vi "gScript Pattern Recognition Tuner.vi"() -> ()   [LabVIEW 2023]
doc: "Use this template to build a controller/worker design pattern. The controller loop always executes. It notifies one or more worker loops to execute their code. The worker loop(s) continue executing until they complete, then wait for another notification. Contrast this with the Producer/Consumer pattern in which the consumer loops execute only when they have data in their queue."
uses:
  find_patches parameters.ctl
  find_circles parameters.ctl
  find_rects_parameters.ctl
  find_template parameters.ctl
  Vision.lvlib
panel:
  in  "Fiducial ID":string
  out "Y Resolution":i32
  out "X Resolution":i32
  out "ROI":cluster{"width(mm)":dbl, "height(mm)":dbl} {"height(mm)" format="%#_3f"; "width(mm)" format="%#_3f"}
  in  "shrinkFactor":i32=4
  in  "Go Button":bool
  in  "Debug":bool
  in  "Field of View":cluster{"fieldOfViewX":sgl, "fieldOfViewY":sgl}={"fieldOfViewX"=1.4, "fieldOfViewY"=1.048}
  out "config lines":string
  out "Log":string
  in  "Results":T1(tab)
  out "Patches":T2(array[cluster])
  out "Circles":T3(array[cluster])
  out "rects":T4(array[cluster]) {"x" format="%#_3g"; "y" format="%#_3g"; "width" format="%#_3g"; "height" format="%#_3g"; "angle" format="%#_3g"; "image-x" format="%#_3g"; "image-y" format="%#_3g"}
  out "Matches":T5(array[cluster])
  in  "Sample Image":path
  out "Image":T6(plugin-control)
  in  "Parameters":T1(tab)
  in  "find_patches parameters":T7={"dilateSize"=6, "sizeMin"=0.1, "sizeMax"=0.3, "aspectRatioMin"=0.1, "aspectRatioMax"=1.1, "colorGroups"=2} {"sizeMin" step=0.05}
  in  "find_circles parameters":T8={"minRadius"=0.1, "maxRadius"=1.0, "houghGradientParam1"=100, "houghGradientParam2"=50}
  in  "find_rects parameters":T9={"nominalWidth"=1.0, "nominalHeight"=1.0, "tolerance"=0.5, "pointSelect"=4.0, "allowRotation"=FALSE}
  in  "find_template parameters":T10={"templateBlurFactor"=0, "minConcurrence"=0.0, "templatePath"="C:\\Users\\Caleb\\Desktop\\nebraska-silicon-lab\\pixel-gantry-control\\Example Project\\Data\\reference_images\\BBM_fid_template.png"}
  # "Tips:\n\n  -"
  # "Tips:\n\n  - minRadius & maxRadius\nare in mm"
  # "Tips:\n\n  - \n\npointSelect:\n  0: center\n  1: bottom-left corner\n  2: top-left corner\n  3: top-right corner\n  4: bottom-right corner"
  # "Tips:\n\n  -"
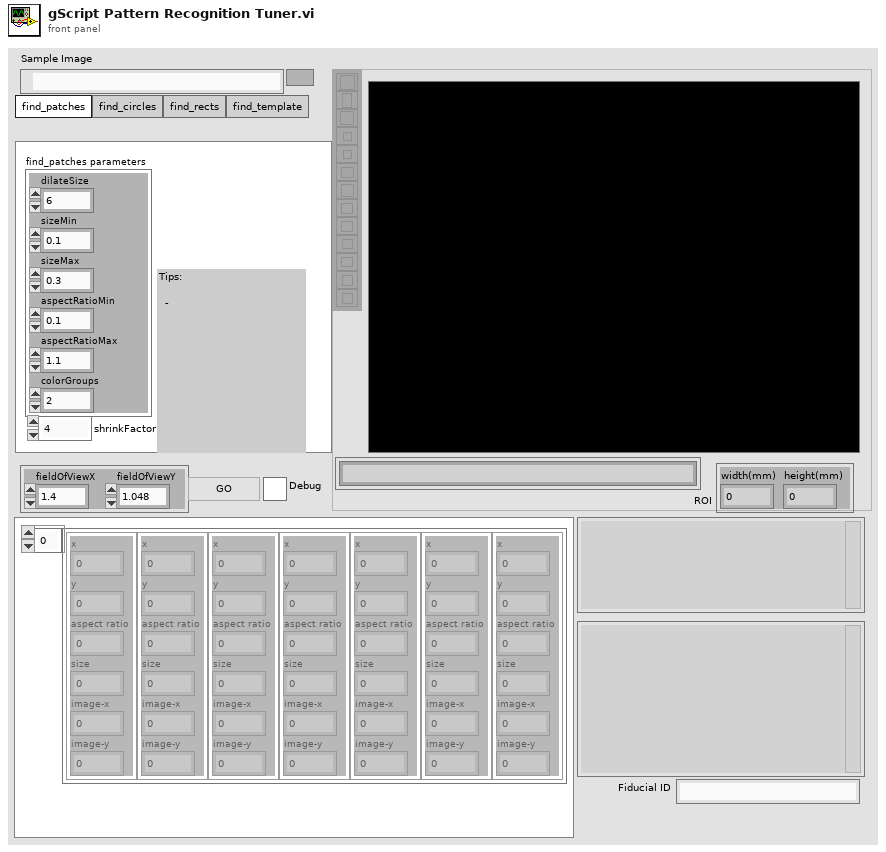
[diagram p1: front panel]
types:
  T1 = enum32{"find_patches", "find_circles", "find_rects", "find_template"}
  T2 = cluster{"x":dbl, "y":dbl, "aspect ratio":dbl, "size":dbl, "image-x":dbl, "image-y":dbl}[]
  T3 = cluster{"x":dbl, "y":dbl, "radius":dbl, "image-x":dbl, "image-y":dbl}[]
  T4 = cluster{"x":dbl, "y":dbl, "width":dbl, "height":dbl, "angle":dbl, "image-x":dbl, "image-y":dbl}[]
  T5 = cluster{"x":dbl, "y":dbl, "image-x":dbl, "image-y":dbl, "Concurrence":dbl}[]
  T6 = typedef "IMAQ Image.ctl" = refnum<image>
  T7 = typedef "Vision.lvlib/find_patches parameters.ctl" = cluster{"dilateSize":i32, "sizeMin":sgl, "sizeMax":sgl, "aspectRatioMin":sgl, "aspectRatioMax":sgl, "colorGroups":i32}
  T8 = typedef "Vision.lvlib/find_circles parameters.ctl" = cluster{"minRadius":sgl, "maxRadius":sgl, "houghGradientParam1":i32, "houghGradientParam2":i32}
  T9 = typedef "Vision.lvlib/find_rects_parameters.ctl" = cluster{"nominalWidth":sgl, "nominalHeight":sgl, "tolerance":sgl, "pointSelect":sgl, "allowRotation":bool}
  T10 = typedef "Vision.lvlib/find_template parameters.ctl" = cluster{"templateBlurFactor":i32, "minConcurrence":sgl, "templatePath":string}
  T11 = enum8{"Enabled", "Disabled", "Disabled and Grayed Out"}
  T12 = cluster{"Left":i32, "Top":i32, "Right":i32, "Bottom":i32}
  T13 = typedef "Image Type" = u32
  T14 = cluster{"Global Rectangle":i32[], "Contours":cluster{"Contour Type":u32, "ROI Type":u32, "Points":i32[]}[]}
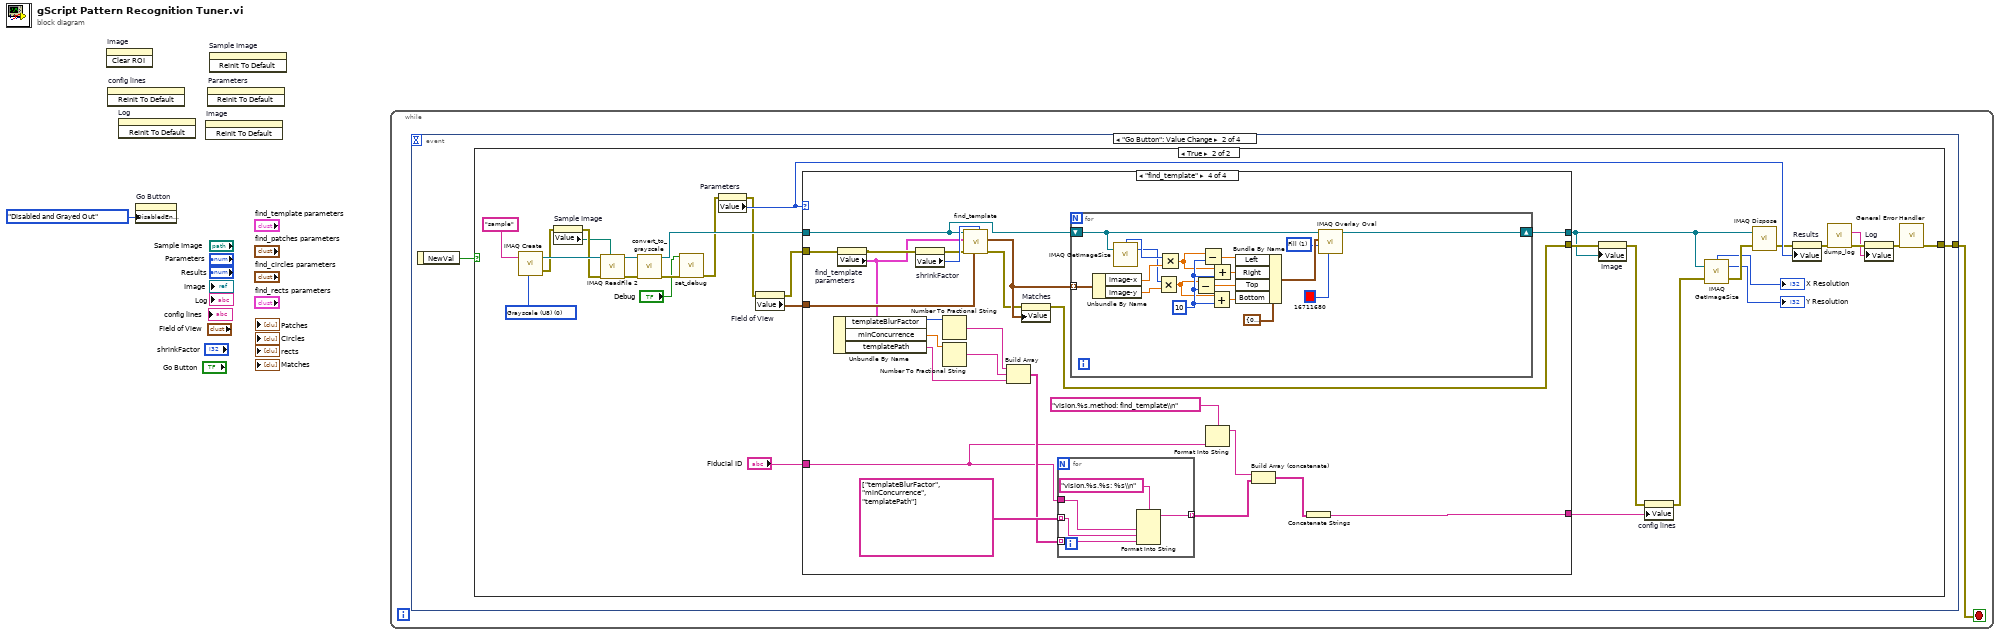
[diagram p0: block diagram]
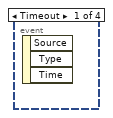
[diagram p2: hidden frame]
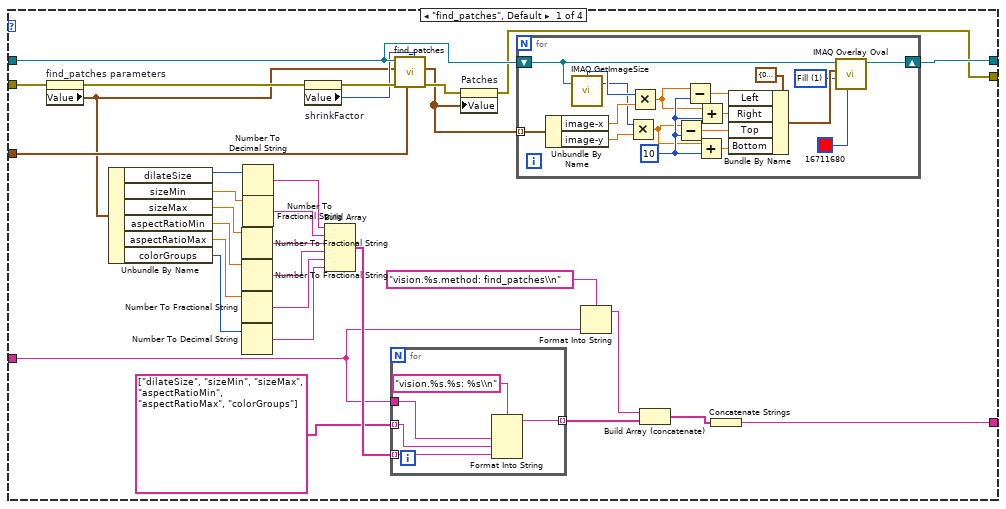
[diagram p4: hidden frame]
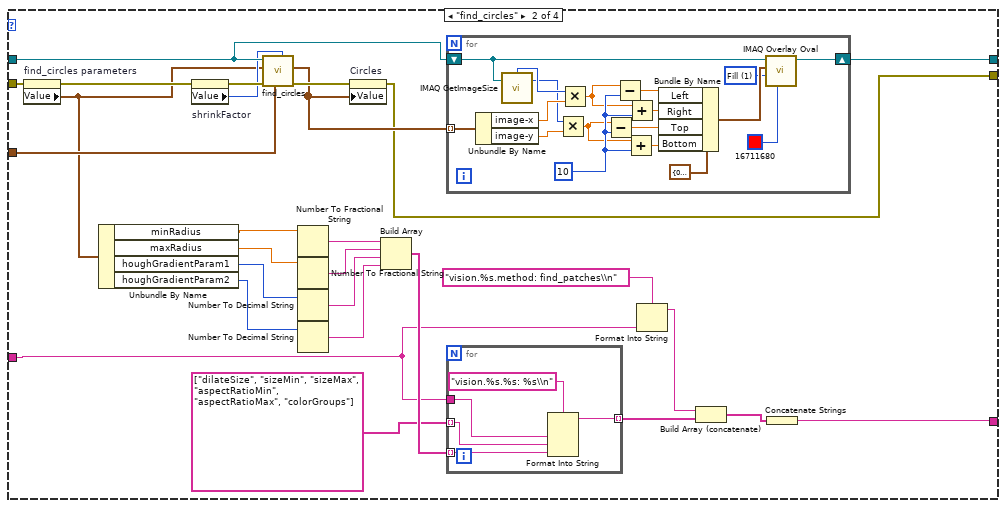
[diagram p5: hidden frame]
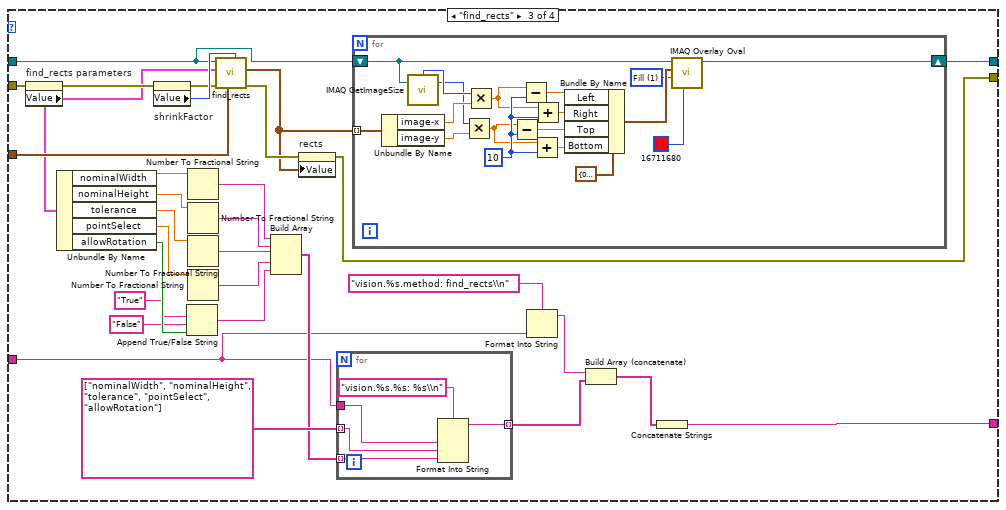
[diagram p6: hidden frame]
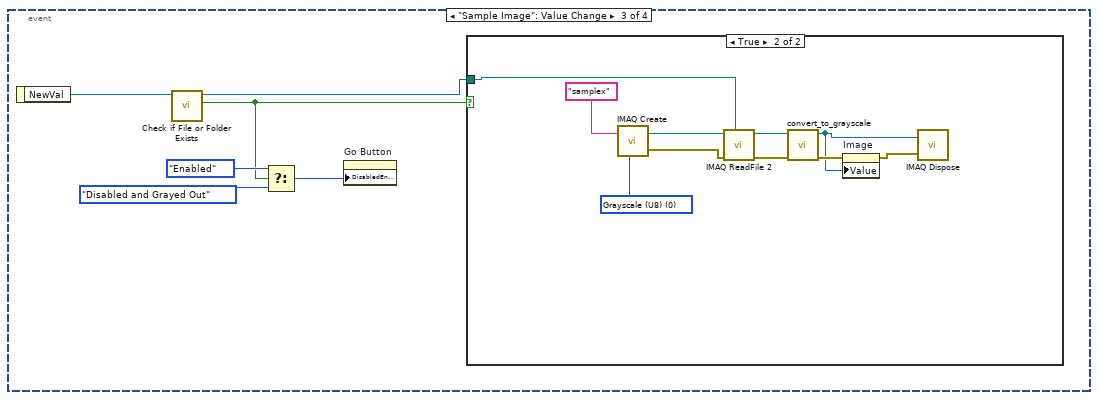
[diagram p7: hidden frame]
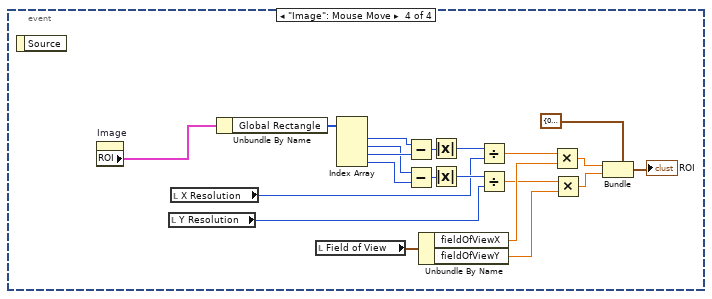
[diagram p9: hidden frame]
diagram:
  n1 = invoke on="Image" class="ImageControl" method="Clear ROI"() -> ()  [unwired: 3 in, 3 out]
  n2 = invoke on="config lines" class="Str" method="Reinit To Default"() -> ()  [unwired: 3 in, 3 out]
  n3 = invoke on="Log" class="Str" method="Reinit To Default"() -> ()  [unwired: 3 in, 3 out]
  n4 = property on="Go Button" class="Bool (strict)"("DisabledEnum"=T11."Disabled and Grayed Out" ("Disabled")) -> ()  [unwired: 2 in, 2 out]
  n5 = invoke on="Image" class="ImageControl" method="Reinit To Default"() -> ()  [unwired: 3 in, 3 out]
  n6 = invoke on="Parameters" class="TabCtl (strict)" method="Reinit To Default"() -> ()  [unwired: 3 in, 3 out]
  n7 = invoke on="Sample Image" class="Path" method="Reinit To Default"() -> ()  [unwired: 3 in, 3 out]
  n8 = while {
    stop <- w2 stop-if-true
    n9 = event shown="[1] \"Go Button\": Value Change" {
      selector: _ -> [_ _ _ _]
      dyn-events: _ -> [_ _ _ _]
      timeout: _ -> [_ _ _ _]
      tunnel: [_ w4 _ _] -> w2
      event Timeout {
        n10 = event-data() -> ()  [unwired: 1 in, 3 out]
      }
      event "Go Button": Value Change {
        n11 = event-data() -> ("NewVal"=w3:bool)  [unwired: 1 in]
        n12 = case shown="True" w3 {
          tunnel: [_ w26] -> w4
          frame False {
          }
          frame True {
            w25 = T13 0 items=["Grayscale (U8)", "Grayscale (I16)", "Grayscale (SGL)", "Complex (CSG)", "RGB (U32)", "HSL (U32)", "RGB (U64)", "Grayscale (U16)"] ("Image Type")
            n13 = call "IMAQ Create"("Image Name"="sample", "Image Type"=w25) -> ("New Image"=w35:T6, "error out"=w34:errorcluster)  [unwired: 3 in]
            n14 = property on="Sample Image" class="Path"(error in=w34) -> (error out=w33:errorcluster, "Value"=w32:path)  [unwired: 1 in, 1 out]
            n15 = call "IMAQ ReadFile 2"("File Path"=w32, "error in (no error)"=w33, "Image"=w35) -> ("error out"=w30:errorcluster, "Image Out"=w31:T6)  [unwired: 4 in, 3 out]
            n16 = call "convert_to_grayscale.vi"("error in (no error)"=w30, "Image in"=w31) -> ("error out"=w19:errorcluster, "Image out"=w29:T6)  [unwired: 8 in]
            n17 = call "set_debug.vi"("error in (no error)"=w19, "debug"="Debug") -> ("error out"=w18:errorcluster)  [unwired: 9 in]
            n18 = property on="Parameters" class="TabCtl (strict)"(error in=w18) -> (error out=w15:errorcluster, "Value"=w28:T1)  [unwired: 1 in, 1 out]
            n19 = property on="Field of View" class="Clust (strict)"(error in=w15) -> (error out=w14:errorcluster, "Value"=w16:cluster{"fieldOfViewX":sgl, "fieldOfViewY":sgl})  [unwired: 1 in, 1 out]
            n20 = case shown="\"find_template\"" w28 {
              tunnel: w29 -> [w63 w112 w165 w214]
              tunnel: w14 -> [w66 w116 w170 w199]
              tunnel: [w61 w111 w162 w194] -> w13
              tunnel: [w64 w110 w164 w213] -> w12
              tunnel: w16 -> [w45 w115 w166 w215]
              tunnel: [w36 w90 w147 w206] -> w8
              tunnel: "Fiducial ID" -> [w46 w99 w140 w201]
              frame "find_patches", Default {
                n21 = property on="find_patches parameters" class="Clust (strict)"(error in=w66) -> (error out=w60:errorcluster, "Value"=w44:T7)  [unwired: 1 in, 1 out]
                n22 = Unbundle By Name(w44) -> ("dilateSize"=w49:i32, "sizeMin"=w50:sgl, "sizeMax"=w51:sgl, "aspectRatioMin"=w42:sgl, "aspectRatioMax"=w41:sgl, "colorGroups"=w40:i32)
                n23 = Number To Fractional String(number=w51) -> (F-format string=w43:string)  [unwired: 3 in]
                n24 = Number To Fractional String(number=w42) -> (F-format string=w39:string)  [unwired: 3 in]
                n25 = Number To Fractional String(number=w41) -> (F-format string=w38:string)  [unwired: 3 in]
                n26 = Number To Decimal String(number=w40) -> (decimal integer string=w37:string)  [unwired: 1 in]
                n27 = Number To Decimal String(number=w49) -> (decimal integer string=w52:string)  [unwired: 1 in]
                n28 = Number To Fractional String(number=w50) -> (F-format string=w53:string)  [unwired: 3 in]
                n29 = property on="shrinkFactor" class="DigNum (strict)"(error in=w60) -> (error out=w59:errorcluster, "Value"=w58:i32)  [unwired: 1 in, 1 out]
                n30 = Build Array(w52, w53, w43, w39, w38, w37) -> (w54:string[])
                n31 = for {
                  tunnel: string[] ["dilateSize", "sizeMin", "sizeMax", "aspectRatioMin", "aspectRatioMax", "colorGroups"] -> [w70] mode=indexing
                  tunnel: w46 -> [w69]
                  tunnel: [w68] -> w56 mode=indexing
                  tunnel: w54 -> [w67] mode=indexing
                  n32 = Format Into String(format string="vision.%s.%s: %s\\n", w69, w70, w67) -> (resulting string=w68:string)  [unwired: 2 in, 1 out]
                }
                n33 = call "find_patches.vi"("Shrink Factor"=w58, "Field of View"=w45, "error in"=w59, "find_patches parameters"=w44, "Image"=w63) -> ("error out"=w65:errorcluster, "Patches"=w62:T2)  [unwired: 5 in]
                n34 = property on="Patches" class="Arr (strict)"(error in=w65, "Value"=w62) -> (error out=w61:errorcluster)  [unwired: 1 in, 1 out]
                n35 = for {
                  tunnel: w62 -> [w89] mode=indexing
                  shift-right: [w73] -> w64
                  shift-left: w63 -> [w84]
                  w72 = u32 1 items=["Frame", "Fill"] ("Drawing Mode (Frame)")
                  w77 = 10
                  n36 = Unbundle By Name(w89) -> ("image-x"=w88:dbl, "image-y"=w86:dbl)
                  n37 = call "IMAQ GetImageSize"("Image"=w84) -> ("Y Resolution"=w85:i32, "X Resolution"=w87:i32)  [unwired: 3 in, 1 out]
                  n38 = Multiply(x=w85, y=w86) -> (x*y=w76:dbl)
                  n39 = Multiply(x=w87, y=w88) -> (x*y=w75:dbl)
                  n40 = Subtract(x=w76, y=w77) -> (x-y=w78:dbl)
                  n41 = Subtract(x=w75, y=w77) -> (x-y=w79:dbl)
                  n42 = Add(x=w76, y=w77) -> (x+y=w80:dbl)
                  n43 = Add(x=w75, y=w77) -> (x+y=w81:dbl)
                  n44 = Bundle By Name(cluster=T12 {"Left"=0, "Top"=0, "Right"=0, "Bottom"=0} ("Bounding Rectangle"), "Left"=w79, "Right"=w81, "Top"=w78, "Bottom"=w80) -> (w74:T12)
                  n45 = call "IMAQ Overlay Oval"("Color"=u32 16711680, "Drawing Mode (Frame)"=w72, "Bounding Rectangle"=w74, "Image"=w84) -> ("Image Out"=w73:T6)  [unwired: 6 in, 1 out]
                }
                n46 = Format Into String(format string="vision.%s.method: find_patches\\n", w46) -> (resulting string=w55:string)  [unwired: 2 in, 1 out]
                n47 = Build Array (concatenate)(w55, w56) -> (w57:string[])
                n48 = Concatenate Strings(w57) -> (w36:string)
              }
              frame "find_circles" {
                n49 = property on="find_circles parameters" class="Clust (strict)"(error in=w116) -> (error out=w109:errorcluster, "Value"=w100:T8)  [unwired: 1 in, 1 out]
                n50 = Unbundle By Name(w100) -> ("minRadius"=w98:sgl, "maxRadius"=w97:sgl, "houghGradientParam1"=w96:i32, "houghGradientParam2"=w95:i32)
                n51 = property on="shrinkFactor" class="DigNum (strict)"(error in=w109) -> (error out=w108:errorcluster, "Value"=w107:i32)  [unwired: 1 in, 1 out]
                n52 = call "find_circles.vi"("shrinkFactor"=w107, "Field of View"=w115, "error in"=w108, "find_circles parameters"=w100, "Image"=w112) -> ("error out"=w114:errorcluster, "Circles"=w113:T3)  [unwired: 5 in]
                n53 = Number To Fractional String(number=w98) -> (F-format string=w94:string)  [unwired: 3 in]
                n54 = Number To Fractional String(number=w97) -> (F-format string=w93:string)  [unwired: 3 in]
                n55 = Number To Decimal String(number=w96) -> (decimal integer string=w92:string)  [unwired: 1 in]
                n56 = Number To Decimal String(number=w95) -> (decimal integer string=w91:string)  [unwired: 1 in]
                n57 = property on="Circles" class="Arr (strict)"(error in=w114, "Value"=w113) -> (error out=w111:errorcluster)  [unwired: 1 in, 1 out]
                n58 = Build Array(w94, w93, w92, w91) -> (w106:string[])
                n59 = for {
                  tunnel: w113 -> [w139] mode=indexing
                  shift-right: [w123] -> w110
                  shift-left: w112 -> [w134]
                  w122 = u32 1 items=["Frame", "Fill"] ("Drawing Mode (Frame)")
                  w127 = 10
                  n60 = Unbundle By Name(w139) -> ("image-x"=w138:dbl, "image-y"=w136:dbl)
                  n61 = call "IMAQ GetImageSize"("Image"=w134) -> ("Y Resolution"=w135:i32, "X Resolution"=w137:i32)  [unwired: 3 in, 1 out]
                  n62 = Multiply(x=w135, y=w136) -> (x*y=w126:dbl)
                  n63 = Multiply(x=w137, y=w138) -> (x*y=w125:dbl)
                  n64 = Subtract(x=w126, y=w127) -> (x-y=w128:dbl)
                  n65 = Subtract(x=w125, y=w127) -> (x-y=w129:dbl)
                  n66 = Add(x=w126, y=w127) -> (x+y=w130:dbl)
                  n67 = Add(x=w125, y=w127) -> (x+y=w131:dbl)
                  n68 = Bundle By Name(cluster=T12 {"Left"=0, "Top"=0, "Right"=0, "Bottom"=0} ("Bounding Rectangle"), "Left"=w129, "Right"=w131, "Top"=w128, "Bottom"=w130) -> (w124:T12)
                  n69 = call "IMAQ Overlay Oval"("Color"=u32 16711680, "Drawing Mode (Frame)"=w122, "Bounding Rectangle"=w124, "Image"=w134) -> ("Image Out"=w123:T6)  [unwired: 6 in, 1 out]
                }
                n70 = for {
                  tunnel: string[] ["dilateSize", "sizeMin", "sizeMax", "aspectRatioMin", "aspectRatioMax", "colorGroups"] -> [w120] mode=indexing
                  tunnel: w99 -> [w119]
                  tunnel: [w118] -> w104 mode=indexing
                  tunnel: w106 -> [w117] mode=indexing
                  n71 = Format Into String(format string="vision.%s.%s: %s\\n", w119, w120, w117) -> (resulting string=w118:string)  [unwired: 2 in, 1 out]
                }
                n72 = Format Into String(format string="vision.%s.method: find_patches\\n", w99) -> (resulting string=w105:string)  [unwired: 2 in, 1 out]
                n73 = Build Array (concatenate)(w105, w104) -> (w103:string[])
                n74 = Concatenate Strings(w103) -> (w90:string)
              }
              frame "find_rects" {
                n75 = property on="find_rects parameters" class="Clust (strict)"(error in=w170) -> (error out=w169:errorcluster, "Value"=w160:T9)  [unwired: 1 in, 1 out]
                n76 = Unbundle By Name(w160) -> ("nominalWidth"=w158:sgl, "nominalHeight"=w157:sgl, "tolerance"=w156:sgl, "pointSelect"=w155:sgl, "allowRotation"=w154:bool)
                n77 = property on="shrinkFactor" class="DigNum (strict)"(error in=w169) -> (error out=w167:errorcluster, "Value"=w168:i32)  [unwired: 1 in, 1 out]
                n78 = Append True/False String(1:w154, 2:"False" ("false string"), 3:"True" ("true string")) -> (0:w149:string)  [unwired: 1 in]
                n79 = Number To Fractional String(number=w158) -> (F-format string=w153:string)  [unwired: 3 in]
                n80 = Number To Fractional String(number=w157) -> (F-format string=w152:string)  [unwired: 3 in]
                n81 = Number To Fractional String(number=w156) -> (F-format string=w151:string)  [unwired: 3 in]
                n82 = Number To Fractional String(number=w155) -> (F-format string=w150:string)  [unwired: 3 in]
                n83 = call "find_rects.vi"("shrinkFactor"=w168, "Field of View"=w166, "error in"=w167, "find_patches parameters"=w160, "Image"=w165) -> ("error out"=w163:errorcluster, "rects"=w161:T4)  [unwired: 5 in]
                n84 = Build Array(w153, w152, w151, w150, w149) -> (w148:string[])
                n85 = property on="rects" class="Arr (strict)"(error in=w163, "Value"=w161) -> (error out=w162:errorcluster)  [unwired: 1 in, 1 out]
                n86 = for {
                  tunnel: string[] ["nominalWidth", "nominalHeight", "tolerance", "pointSelect", "allowRotation"] -> [w174] mode=indexing
                  tunnel: w140 -> [w173]
                  tunnel: [w172] -> w142 mode=indexing
                  tunnel: w148 -> [w171] mode=indexing
                  n87 = Format Into String(format string="vision.%s.%s: %s\\n", w173, w174, w171) -> (resulting string=w172:string)  [unwired: 2 in, 1 out]
                }
                n88 = for {
                  shift-right: [w178] -> w164
                  shift-left: w165 -> [w189]
                  tunnel: w161 -> [w176] mode=indexing
                  w177 = u32 1 items=["Frame", "Fill"] ("Drawing Mode (Frame)")
                  w182 = 10
                  n89 = Unbundle By Name(w176) -> ("image-x"=w193:dbl, "image-y"=w191:dbl)
                  n90 = call "IMAQ GetImageSize"("Image"=w189) -> ("Y Resolution"=w190:i32, "X Resolution"=w192:i32)  [unwired: 3 in, 1 out]
                  n91 = Multiply(x=w190, y=w191) -> (x*y=w181:dbl)
                  n92 = Multiply(x=w192, y=w193) -> (x*y=w180:dbl)
                  n93 = Subtract(x=w181, y=w182) -> (x-y=w183:dbl)
                  n94 = Subtract(x=w180, y=w182) -> (x-y=w184:dbl)
                  n95 = Add(x=w181, y=w182) -> (x+y=w185:dbl)
                  n96 = Add(x=w180, y=w182) -> (x+y=w186:dbl)
                  n97 = Bundle By Name(cluster=T12 {"Left"=0, "Top"=0, "Right"=0, "Bottom"=0} ("Bounding Rectangle"), "Left"=w184, "Right"=w186, "Top"=w183, "Bottom"=w185) -> (w179:T12)
                  n98 = call "IMAQ Overlay Oval"("Color"=u32 16711680, "Drawing Mode (Frame)"=w177, "Bounding Rectangle"=w179, "Image"=w189) -> ("Image Out"=w178:T6)  [unwired: 6 in, 1 out]
                }
                n99 = Format Into String(format string="vision.%s.method: find_rects\\n", w140) -> (resulting string=w143:string)  [unwired: 2 in, 1 out]
                n100 = Build Array (concatenate)(w143, w142) -> (w141:string[])
                n101 = Concatenate Strings(w141) -> (w147:string)
              }
              frame "find_template" {
                n102 = property on="find_template parameters" class="Clust (strict)"(error in=w199) -> (error out=w198:errorcluster, "Value"=w197:T10)  [unwired: 1 in, 1 out]
                n103 = Unbundle By Name(w197) -> ("templateBlurFactor"=w211:i32, "minConcurrence"=w210:sgl, "templatePath"=w200:string)
                n104 = property on="shrinkFactor" class="DigNum (strict)"(error in=w198) -> (error out=w216:errorcluster, "Value"=w217:i32)  [unwired: 1 in, 1 out]
                n105 = Number To Fractional String(number=w211) -> (F-format string=w209:string)  [unwired: 3 in]
                n106 = Number To Fractional String(number=w210) -> (F-format string=w208:string)  [unwired: 3 in]
                n107 = call "find_template.vi"("Shrink Factor"=w217, "Field of View"=w215, "error in"=w216, "find_template parameters"=w197, "Image"=w214) -> ("error out"=w195:errorcluster, "Matches"=w196:T5)  [unwired: 5 in]
                n108 = Build Array(w209, w208, w200) -> (w207:string[])
                n109 = property on="Matches" class="Arr (strict)"(error in=w195, "Value"=w196) -> (error out=w194:errorcluster)  [unwired: 1 in, 1 out]
                n110 = for {
                  tunnel: string[] ["templateBlurFactor", "minConcurrence", "templatePath"] -> [w221] mode=indexing
                  tunnel: w201 -> [w220]
                  tunnel: [w219] -> w203 mode=indexing
                  tunnel: w207 -> [w218] mode=indexing
                  n111 = Format Into String(format string="vision.%s.%s: %s\\n", w220, w221, w218) -> (resulting string=w219:string)  [unwired: 2 in, 1 out]
                }
                n112 = for {
                  shift-right: [w225] -> w213
                  shift-left: w214 -> [w236]
                  tunnel: w196 -> [w223] mode=indexing
                  w224 = u32 1 items=["Frame", "Fill"] ("Drawing Mode (Frame)")
                  w229 = 10
                  n113 = Unbundle By Name(w223) -> ("image-x"=w240:dbl, "image-y"=w238:dbl)
                  n114 = call "IMAQ GetImageSize"("Image"=w236) -> ("Y Resolution"=w237:i32, "X Resolution"=w239:i32)  [unwired: 3 in, 1 out]
                  n115 = Multiply(x=w237, y=w238) -> (x*y=w228:dbl)
                  n116 = Multiply(x=w239, y=w240) -> (x*y=w227:dbl)
                  n117 = Subtract(x=w228, y=w229) -> (x-y=w230:dbl)
                  n118 = Subtract(x=w227, y=w229) -> (x-y=w231:dbl)
                  n119 = Add(x=w228, y=w229) -> (x+y=w232:dbl)
                  n120 = Add(x=w227, y=w229) -> (x+y=w233:dbl)
                  n121 = Bundle By Name(cluster=T12 {"Left"=0, "Top"=0, "Right"=0, "Bottom"=0} ("Bounding Rectangle"), "Left"=w231, "Right"=w233, "Top"=w230, "Bottom"=w232) -> (w226:T12)
                  n122 = call "IMAQ Overlay Oval"("Color"=u32 16711680, "Drawing Mode (Frame)"=w224, "Bounding Rectangle"=w226, "Image"=w236) -> ("Image Out"=w225:T6)  [unwired: 6 in, 1 out]
                }
                n123 = Format Into String(format string="vision.%s.method: find_template\\n", w201) -> (resulting string=w204:string)  [unwired: 2 in, 1 out]
                n124 = Build Array (concatenate)(w204, w203) -> (w202:string[])
                n125 = Concatenate Strings(w202) -> (w206:string)
              }
            }
            n126 = property on="Image" class="ImageControl"(error in=w13, "Value"=w12) -> (error out=w7:errorcluster)  [unwired: 1 in, 1 out]
            n127 = property on="config lines" class="Str"(error in=w7, "Value"=w8) -> (error out=w6:errorcluster)  [unwired: 1 in, 1 out]
            n128 = call "IMAQ GetImageSize"("Image"=w12, "error in (no error)"=w6) -> ("Y Resolution"=→"Y Resolution":i32, "X Resolution"=→"X Resolution":i32, "error out"=w11:errorcluster)  [unwired: 2 in]
            n129 = call "IMAQ Dispose"("Image"=w12, "error in (no error)"=w11) -> ("error out"=w27:errorcluster)  [unwired: 4 in]
            n130 = property on="Results" class="TabCtl (strict)"(error in=w27, "Value"=w28) -> (error out=w23:errorcluster)  [unwired: 1 in, 1 out]
            n131 = call "dump_log.vi"("error in (no error)"=w23) -> ("error out"=w22:errorcluster, "log out"=w21:string)  [unwired: 9 in]
            n132 = property on="Log" class="Str"(error in=w22, "Value"=w21) -> (error out=w20:errorcluster)  [unwired: 1 in, 1 out]
            n133 = call <vilib>:"General Error Handler.vi"("error in (no error)"=w20) -> ("error out"=w26:errorcluster)  [unwired: 10 in, 4 out]
          }
        }
      }
      event "Sample Image": Value Change {
        n134 = event-data() -> ("NewVal"=w246:path)  [unwired: 1 in]
        n135 = call <vilib>:"Check if File or Folder Exists.vi"("path"=w246) -> ("file or folder exists?"=w242:bool, "dup path"=w241:path)  [unwired: 8 in, 1 out]
        n136 = Select(t=T11."Enabled" ("Disabled"), s=w242, f=T11."Disabled and Grayed Out") -> (s? t:f=w243:T11)
        n137 = property on="Go Button" class="Bool (strict)"("DisabledEnum"=w243) -> ()  [unwired: 2 in, 2 out]
        n138 = case shown="True" w242 {
          tunnel: w241 -> [_ w253]
          frame False {
          }
          frame True {
            w256 = T13 0 items=["Grayscale (U8)", "Grayscale (I16)", "Grayscale (SGL)", "Complex (CSG)", "RGB (U32)", "HSL (U32)", "RGB (U64)", "Grayscale (U16)"] ("Image Type")
            n139 = call "IMAQ Create"("Image Name"="samplex", "Image Type"=w256) -> ("New Image"=w254:T6, "error out"=w252:errorcluster)  [unwired: 3 in]
            n140 = call "IMAQ ReadFile 2"("File Path"=w253, "error in (no error)"=w252, "Image"=w254) -> ("error out"=w251:errorcluster, "Image Out"=w250:T6)  [unwired: 4 in, 3 out]
            n141 = call "convert_to_grayscale.vi"("error in (no error)"=w251, "Image in"=w250) -> ("error out"=w249:errorcluster, "Image out"=w247:T6)  [unwired: 8 in]
            n142 = property on="Image" class="ImageControl"(error in=w249, "Value"=w247) -> (error out=w248:errorcluster)  [unwired: 1 in, 1 out]
            n143 = call "IMAQ Dispose"("Image"=w247, "error in (no error)"=w248) -> ()  [unwired: 4 in, 1 out]
          }
        }
      }
      event "Image": Mouse Move {
        n144 = event-data() -> ()  [unwired: 1 in, 1 out]
        n145 = property on="Image" class="ImageControl"() -> ("ROI"=w277:T14)  [unwired: 2 in, 2 out]
        n146 = local read "Y Resolution"() -> (w257:i32)
        n147 = local read "X Resolution"() -> (w258:i32)
        n148 = Unbundle By Name(w277) -> ("Global Rectangle"=w276:i32[])
        n149 = local read "Field of View"() -> (w267:cluster{"fieldOfViewX":sgl, "fieldOfViewY":sgl})
        n150 = Index Array(array=w276) -> (element #1=w273:i32, element #2=w271:i32, element #3=w272:i32, element #4=w270:i32)  [unwired: 4 in]
        n151 = Subtract(x=w273, y=w272) -> (x-y=w275:i32)
        n152 = Subtract(x=w271, y=w270) -> (x-y=w274:i32)
        n153 = Unbundle By Name(w267) -> ("fieldOfViewX"=w265:sgl, "fieldOfViewY"=w263:sgl)
        n154 = Absolute Value(x=w275) -> (abs(x)=w269:i32)
        n155 = Absolute Value(x=w274) -> (abs(x)=w268:i32)
        n156 = Divide(x=w269, y=w258) -> (x/y=w266:dbl)
        n157 = Divide(x=w268, y=w257) -> (x/y=w264:dbl)
        n158 = Multiply(x=w266, y=w265) -> (x*y=w261:dbl)
        n159 = Multiply(x=w264, y=w263) -> (x*y=w260:dbl)
        n160 = Bundle(cluster=cluster{"width(mm)":dbl, "height(mm)":dbl} {"width(mm)"=0.0, "height(mm)"=0.0} ("ROI"), "width(mm)"=w261, "height(mm)"=w260) -> (→"ROI":cluster{"width(mm)":dbl, "height(mm)":dbl})
      }
    }
  }
